vi "pulses2_commands_T2.vi"(10 "Dark_time_us":dbl, 11 "T2_parameters":T1) -> (2 "Sequence_time_us":dbl format="%#_13g", 3 "Array out":T2(array[cluster]))   [LabVIEW 2014]
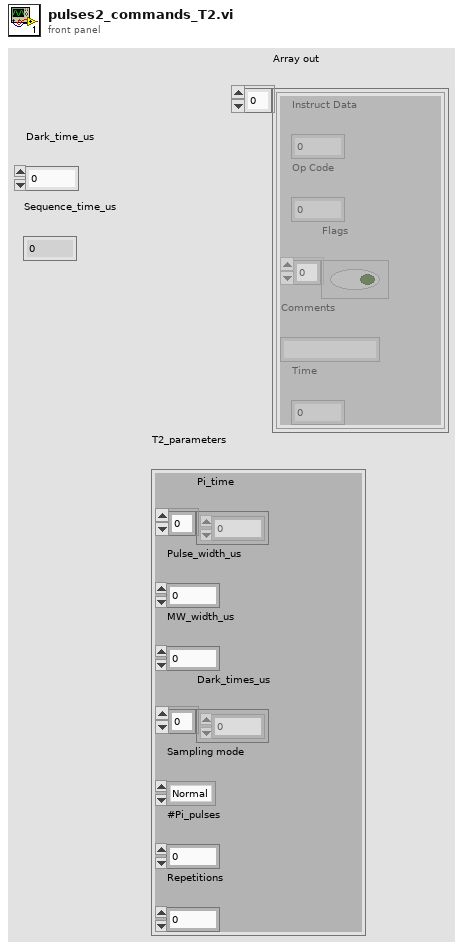
[diagram p1: front panel]
types:
  T1 = cluster{"Pi_time":dbl[], "Pulse_width_us":dbl, "MW_width_us":dbl, "Dark_times_us":dbl[], "Sampling mode":enum16{"Normal", "Sweep"}, "#Pi_pulses":i32, "Repetitions":i32}
  T2 = cluster{"Instruct Data":i32, "Op Code":i32, "Flags":bool[], "Comments":string, "Time":dbl}[]
  T3 = cluster{"Instruct Data":i32, "Op Code":i32, "Flags":bool[], "Comments":string, "Time":dbl}
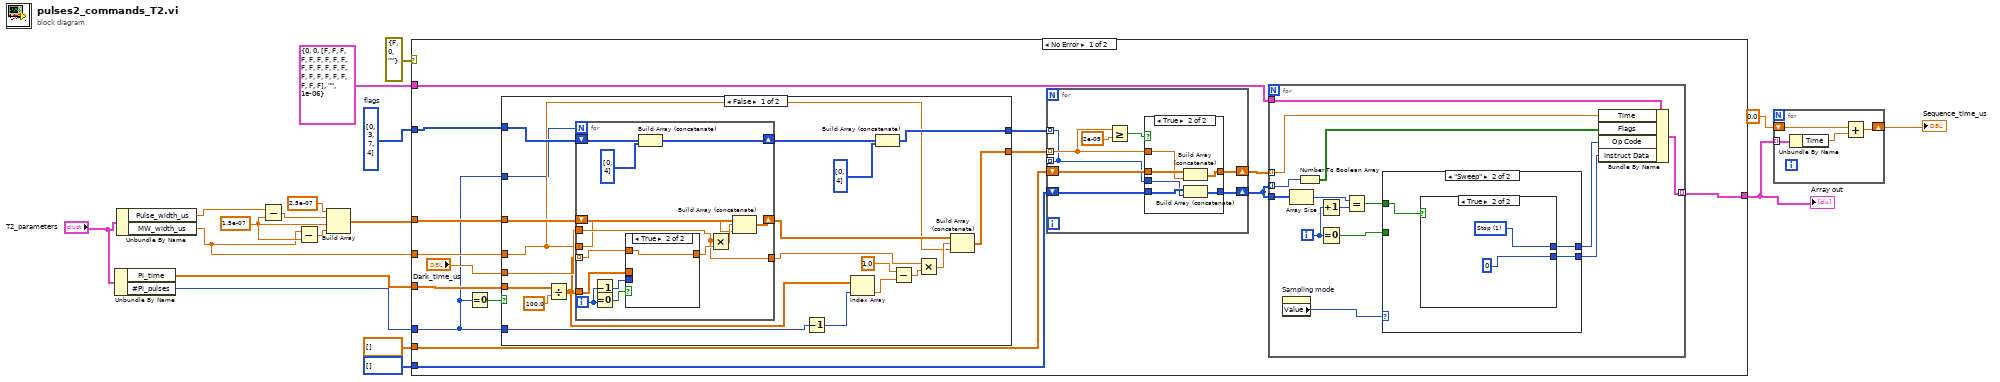
[diagram p0: block diagram]
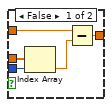
[diagram p2: hidden frame]
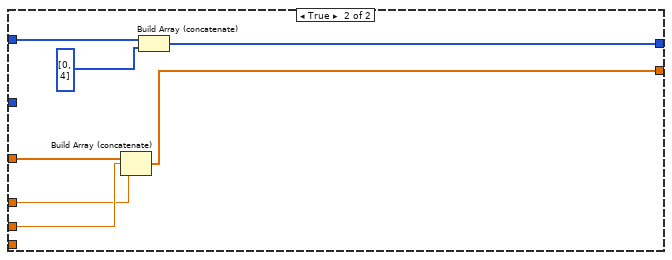
[diagram p3: hidden frame]
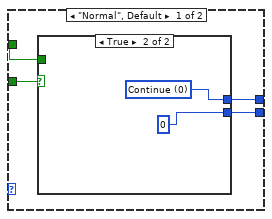
[diagram p4: hidden frame]
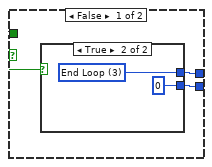
[diagram p5: hidden frame]
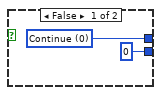
[diagram p6: hidden frame]
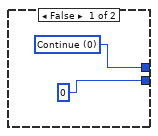
[diagram p7: hidden frame]
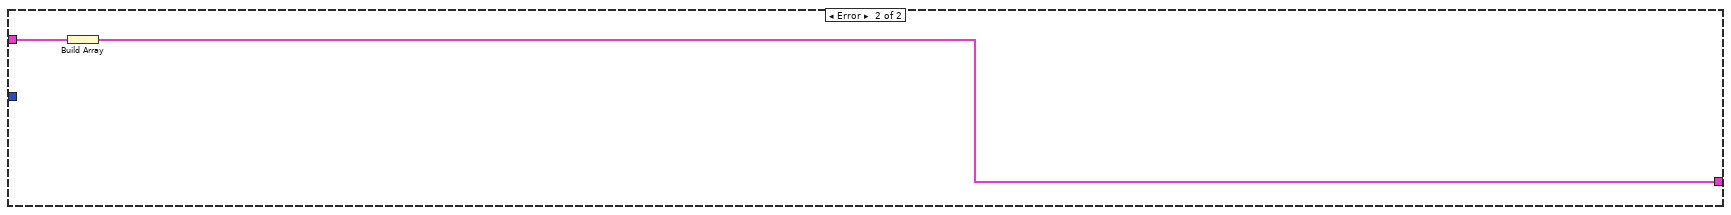
[diagram p9: hidden frame]
diagram:
  w14 = 1.5e-07
  w10 = u8[] [0, 3, 7, 4]  # flags
  n1 = Unbundle By Name("T2_parameters") -> ("Pi_time"=w5:dbl[], "#Pi_pulses"=w4:i32)
  n2 = Unbundle By Name("T2_parameters") -> ("Pulse_width_us"=w8:dbl, "MW_width_us"=w7:dbl)
  n3 = Subtract(x=w8, y=w14) -> (x-y=w12:dbl)
  n4 = Subtract(x=w7, y=w14) -> (x-y=w15:dbl)
  n5 = Build Array(2.5e-07, w12, w14, w15) -> (w11:dbl[])
  n6 = case shown="No Error" errorcluster {"status"=FALSE, "code"=0, "source"=""} ("error constant") {
    tunnel: w11 -> [w27 _]
    tunnel: dbl[] [] -> [w33 _]
    tunnel: u8[] [] -> [w32 _]
    tunnel: w10 -> [w26 _]
    tunnel: T3 {"Instruct Data"=0, "Op Code"=0, "Flags"=[FALSE, FALSE, FALSE, FALSE, FALSE, FALSE, FALSE, FALSE, FALSE, FALSE, FALSE, FALSE, FALSE, FALSE, FALSE, FALSE, FALSE, FALSE, FALSE, FALSE, FALSE, FALSE, FALSE, FALSE], "Comments"="", "Time"=1e-06} ("PB Instruction") -> [w31 w131]
    tunnel: [w19 w132] -> w2
    tunnel: w7 -> [w25 _]
    tunnel: w5 -> [w21 _]
    tunnel: w4 -> [w20 _]
    frame No Error {
      n7 = Equal To 0?(x=w20) -> (x = 0?=w28:bool)
      n8 = case shown="False" w28 {
        tunnel: w27 -> [w50 w78]
        tunnel: w26 -> [w49 w80]
        tunnel: w25 -> [w38 w76]
        tunnel: "Dark_time_us" -> [w51 w77]
        tunnel: [w42 w75] -> w23
        tunnel: [w39 w74] -> w22
        tunnel: w21 -> [w53 _]
        tunnel: w20 -> [w36 _]
        tunnel: w20 -> [w34 _]
        frame False {
          n9 = Divide(x=w53, y=100.0) -> (x/y=w37:dbl[])
          n10 = for {
            N: w34 -> [_]
            tunnel: w37 -> [w66]
            tunnel: w37 -> [w63] mode=indexing
            tunnel: w51 -> [w55]
            shift-right: [w59] -> w43
            shift-left: w50 -> [w60]
            shift-right: [w56] -> w40
            shift-left: w49 -> [w58]
            tunnel: [w55] -> w45
            tunnel: w38 -> [w54]
            i -> [w65]
            n11 = Decrement(x=w65) -> (x-1=w64:i32)
            n12 = Equal To 0?(x=w65) -> (x = 0?=w67:bool)
            n13 = case shown="True" w67 {
              tunnel: w66 -> [w72 _]
              tunnel: w64 -> [w71 _]
              tunnel: w63 -> [w69 w73]
              tunnel: [w68 w73] -> w62
              frame False {
                n14 = Index Array(array=w72, index=w71) -> (element=w70:dbl)
                n15 = Subtract(x=w69, y=w70) -> (x-y=w68:dbl)
              }
              frame True {
              }
            }
            n16 = Build Array (concatenate)(w58, i32[] [0, 4]) -> (w56:i32[])
            n17 = Multiply(x=w55, y=w62) -> (x*y=w61:dbl)
            n18 = Build Array (concatenate)(w60, w61, w54) -> (w59:dbl[])
          }
          n19 = Decrement(x=w36) -> (x-1=w35:i32)
          n20 = Index Array(array=w37, index=w35) -> (element=w48:dbl)
          n21 = Build Array (concatenate)(w40, i32[] [0, 4]) -> (w39:i32[])
          n22 = Subtract(x=1.0, y=w48) -> (x-y=w46:dbl)
          n23 = Multiply(x=w45, y=w46) -> (x*y=w44:dbl)
          n24 = Build Array (concatenate)(w43, w44, w38) -> (w42:dbl[])
        }
        frame True {
          n25 = Build Array (concatenate)(w78, w77, w76) -> (w75:dbl[])
          n26 = Build Array (concatenate)(w80, i32[] [0, 4]) -> (w74:i32[])
        }
      }
      n27 = for {
        tunnel: w23 -> [w119] mode=indexing
        shift-right: [w116] -> w29
        shift-left: w32 -> [w118]
        shift-right: [w117] -> w30
        shift-left: w33 -> [w120]
        tunnel: [w115] -> _ mode=indexing
        tunnel: w22 -> [w115] mode=indexing
        n28 = Greater Or Equal?(x=w119, y=2e-09) -> (x >= y?=w122:bool)
        n29 = case shown="True" w122 {
          tunnel: w120 -> [w124 w130]
          tunnel: w119 -> [_ w129]
          tunnel: w118 -> [w123 w128]
          tunnel: w115 -> [_ w127]
          tunnel: [w124 w126] -> w117
          tunnel: [w123 w125] -> w116
          frame False {
          }
          frame True {
            n30 = Build Array (concatenate)(w130, w129) -> (w126:dbl[])
            n31 = Build Array (concatenate)(w128, w127) -> (w125:i32[])
          }
        }
      }
      n32 = for {
        tunnel: w31 -> [w93]
        tunnel: w30 -> [w85] mode=indexing
        tunnel: w29 -> [w87]
        tunnel: w29 -> [w84] mode=indexing
        tunnel: [w82] -> w19 mode=indexing
        i -> [w88]
        n33 = property on="Sampling mode" class="Enum (strict)"() -> ("Value"=w81:enum16{"Normal", "Sweep"})  [unwired: 2 in, 2 out]
        n34 = Array Size(array=w87) -> (size(s)=w86:i32)
        n35 = Number To Boolean Array(number=w84) -> (Boolean array=w83:bool[])
        n36 = Increment(x=w88) -> (x+1=w89:i32)
        n37 = Equal To 0?(x=w88) -> (x = 0?=w94:bool)
        n38 = Equal?(x=w86, y=w89) -> (x = y?=w90:bool)
        n39 = case shown="\"Sweep\"" w81 {
          tunnel: w94 -> [w98 _]
          tunnel: [w97 w108] -> w92
          tunnel: [w96 w109] -> w91
          tunnel: w90 -> [w95 w110]
          frame "Normal", Default {
            n40 = case shown="True" w98 {
              tunnel: [w100 0] -> w97
              tunnel: [w99 w107] -> w96
              tunnel: w95 -> [w101 _]
              frame False {
                n41 = case shown="True" w101 {
                  tunnel: [0 0] -> w100
                  tunnel: [w103 w104] -> w99
                  frame False {
                    w103 = 0 items=["Continue", "Stop", "Loop", "End Loop", "JSR", "RTS", "Branch", "Long Delay", "Wait"] ("Op Code")
                  }
                  frame True {
                    w104 = 3 items=["Continue", "Stop", "Loop", "End Loop", "JSR", "RTS", "Branch", "Long Delay", "Wait"] ("Op Code 2")
                  }
                }
              }
              frame True {
                w107 = 0 items=["Continue", "Stop", "Loop", "End Loop", "JSR", "RTS", "Branch", "Long Delay", "Wait"] ("Op Code 2")
              }
            }
          }
          frame "Sweep" {
            n42 = case shown="True" w110 {
              tunnel: [w112 w114] -> w109
              tunnel: [0 0] -> w108
              frame False {
                w112 = 0 items=["Continue", "Stop", "Loop", "End Loop", "JSR", "RTS", "Branch", "Long Delay", "Wait"] ("Op Code 2")
              }
              frame True {
                w114 = 1 items=["Continue", "Stop", "Loop", "End Loop", "JSR", "RTS", "Branch", "Long Delay", "Wait"] ("Op Code 2")
              }
            }
          }
        }
        n43 = Bundle By Name(cluster=w93, "Time"=w85, "Flags"=w83, "Op Code"=w91, "Instruct Data"=w92) -> (w82:T3)
      }
    }
    frame Error {
      n44 = Build Array(w131) -> (w132:T2)
    }
  }
  "Array out" <- w2
  n45 = for {
    shift-right: [w133] -> w1
    shift-left: 0.0 -> [w134]
    tunnel: w2 -> [w136] mode=indexing
    n46 = Unbundle By Name(w136) -> ("Time"=w135:dbl)
    n47 = Add(x=w134, y=w135) -> (x+y=w133:dbl)
  }
  "Sequence_time_us" <- w1
